vi "RRTPlan.vi"(4 "AttackerAvoidArea":bool=TRUE, 5 "Parameters.lvclass":refnum<class "Parameters.lvclass">, 6 "Line?":bool, 7 "Volta ao redor\nda área?":bool, 8 "Initial Pos x,y":dbl[](array[numeric]), 9 "Dest x,y":dbl[](array[numeric]), 10 "IA State":T1={"our_robots"=[], "enemy_robots"=[], "balls"=[], "geometry"={"line_width"=0, "field_length"=0, "field_width"=0, "boundary_width"=0, "referee_width"=0, "goal_width"=0, "goal_depth"=0, "goal_wall_width"=0, "center_circle_radius"=0, "defense_radius"=0, "defense_stretch"=0, "free_kick_from_defense_dist"=0, "penalty_spot_from_field_line_dist"=0, "penalty_line_from_spot_dist"=0}, "IA Judge"={"stage"="", "command"="", "our_goalie_id"=0.0, "enemy_goalie_id"=0.0, "command enum"=enum."Halt", "Time"=enum."Azul", "Point"={"x"=0.0, "y"=0.0}}, "Received Timestamp"=timestamp(0 s since 1904-01-01), "Events"={"Touch"=FALSE, "Ball out"=FALSE, "id touch"=0.0, "Ball out of \nVision"=FALSE, "Ball inside \nGoalie area"=FALSE, "Robot not responding"=FALSE, "Robots responding status"=[1.0, 1.0, 1.0, 1.0, 1.0, 1.0], "Enemy Ball \nPossession"=FALSE, "Pass State"=FALSE, "id end of pass"=0.0, "Kick"=FALSE, "Id ini Possession"=0.0, "Ball Possesion"=FALSE, "Id Possesion"=0.0, "Direct Kick"=FALSE, "2nd Strk Ativo"=FALSE}}, 11 "Robot":T2={"id"=0, "function"=enum."Attacker", "x"=0.0, "y"=0.0, "orientation"=0.0, "v_tangent"=0.0, "v_normal"=0.0, "v_ang"=0.0, "kick_x"=0.0, "kick_z"=0.0, "dribble"=FALSE, "Timestamp"=timestamp(0 s since 1904-01-01), "estimatives"={"est_v_tangent"=0.0, "est_v_normal"=0.0, "est_vx"=0.0, "est_vy"=0.0, "Pos Robot Est"=[], "est_v_ang"=0.0}, "dest_x_kick"=0.0, "dest_y_kick"=0.0, "Gap Coord"=[], "States"=enum."GoToTangent", "Path "=[], "Path  Smooth"=[], "Dest"=[], "vx_desired"=0.0, "vy_desired"=0.0, "slowBehavior"=FALSE, "VSSStates"=enum."Pass", "robotKickState"=enum."none", "role"=enum."DefenderArea"}) -> (0 "Path":dbl[][](array[numeric]), 1 "Smooth Path":dbl[][](array[numeric]))   [LabVIEW 2020]
uses:
  Vision_class/Old vision/Controls/AI Robot.ctl
  Vision_class/Old vision/Controls/Functions Enum.ctl
  Controls/estimatives.ctl
  Vision_class/Old vision/Controls/AttackerStates.ctl
  Vision_class/Old vision/Controls/PathDests.ctl
  Vision_class/Old vision/Controls/PathDest.ctl
  Navigation/VSSNavigation/VSSAttackerStates.ctl
  Robot_class/robotKickToStates.ctl
  Robot_class/roles.ctl
  Vision_class/Old vision/SSL Detection Frame Simple Estimator Cameras VelCmd Folder/Core/AI Input.ctl
  Vision_class/Old vision/SSL Detection Frame Simple Estimator Cameras VelCmd Folder/Core/AI Ball.ctl
  Vision_class/Old vision/SSL Detection Frame Simple Estimator Cameras VelCmd Folder/Core/Field Size.ctl
  Vision_class/Old vision/SSL Detection Frame Simple Estimator Cameras VelCmd Folder/Core/AI Judge.ctl
  Communication_class/Paths/MessageAI_State Folder/Intel/Command Enum.ctl
  Vision_class/Old vision/SSL Detection Frame Simple Estimator Cameras VelCmd Folder/Util/Events/Events.ctl
  Parameters_class/Parameters.lvclass
  Utilities_class/Utilities.lvclass
  Parameters_class/Parameters.lvclass/Parameters.ctl
  <vilib>/Analysis/_algsub.llb/Real Vector Norm.vi
  Parameters_class/Read Project.vi
  <vilib>/Analysis/NI_AALPro.lvlib
panel:
  in  "Path out":dbl[][](array[numeric])
  out "Path out 2":dbl[][](array[numeric])
  in  "WayPointProb":dbl=0.6 format="%#_13g"
  in  "GoalProb":dbl=0.1 format="%#_13g"
  in  "Step":dbl=80.0
  out "Goal":dbl[](array[numeric])
  out "Initial State":dbl[](array[numeric])
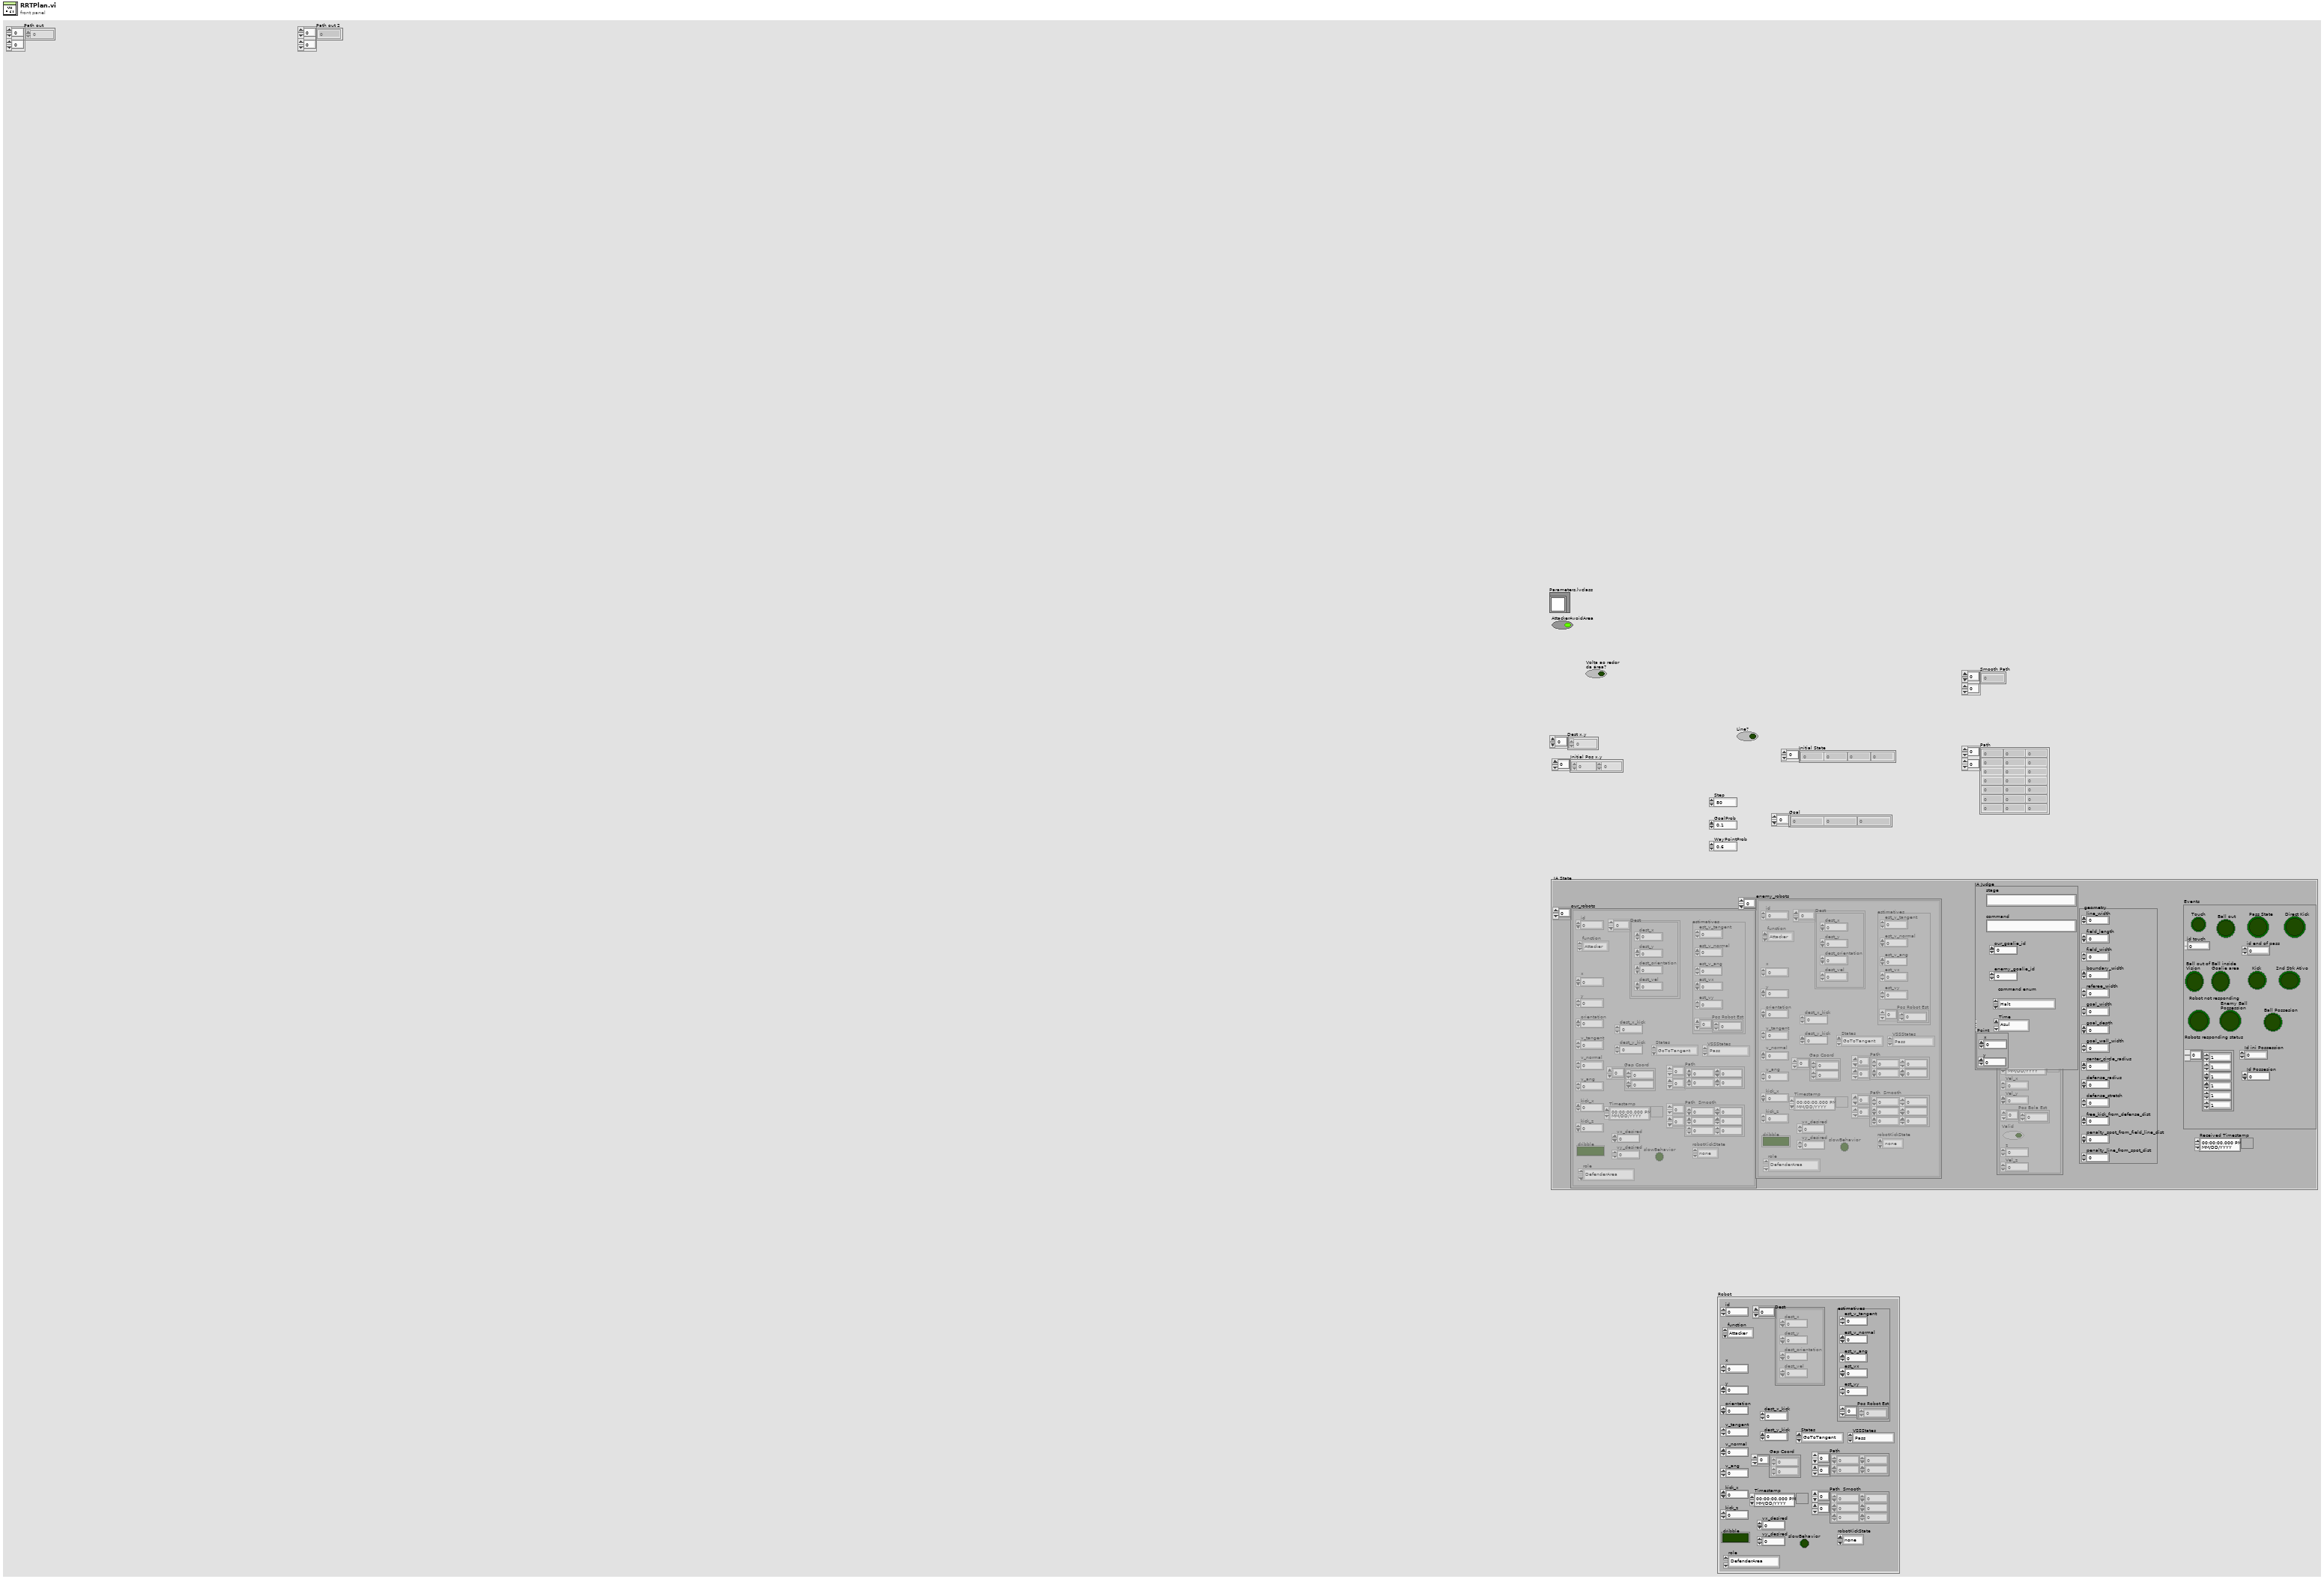
[diagram p1: front panel]
types:
  T1 = typedef "AI Input.ctl" = cluster{"our_robots":T2[], "enemy_robots":T2[], "balls":T11[], "geometry":T12, "IA Judge":T13, "Received Timestamp":timestamp, "Events":T15}
  T2 = typedef "AI Robot.ctl" = cluster{"id":u32, "function":T3, "x":dbl, "y":dbl, "orientation":dbl, "v_tangent":dbl, "v_normal":dbl, "v_ang":dbl, "kick_x":dbl, "kick_z":dbl, "dribble":bool, "Timestamp":timestamp, "estimatives":T4, "dest_x_kick":dbl, "dest_y_kick":dbl, "Gap Coord":dbl[], "States":T5, "Path ":dbl[][], "Path  Smooth":dbl[][], "Dest":T6, "vx_desired":dbl, "vy_desired":dbl, "slowBehavior":bool, "VSSStates":T8, "robotKickState":T9, "role":T10}
  T3 = typedef "Functions Enum.ctl" = enum16{"2nd Striker", "Attacker", "Goalie", "Defender", "Striker", "Goto 0", "Dummy", "Kicker", "ZigZag 0", "ZigZag 1", "ZigZag 2", "ZigZag 3", "ZigZag 4", "ZigZag 5", "ZigZag 6", "ZigZag 7", "ZigZag 8", ""}
  T4 = typedef "estimatives.ctl" = cluster{"est_v_tangent":dbl, "est_v_normal":dbl, "est_vx":dbl, "est_vy":dbl, "Pos Robot Est":dbl[], "est_v_ang":dbl}
  T5 = typedef "AttackerStates.ctl" = enum16{"Pass", "GoToTangent", "BallGetting", "GoToKick", ""}
  T6 = typedef "PathDests.ctl" = T7[]
  T7 = typedef "PathDest.ctl" = cluster{"dest_x":dbl, "dest_y":dbl, "dest_orientation":dbl, "dest_vel":dbl}
  T8 = typedef "VSSAttackerStates.ctl" = enum16{"Pass", "GoToTangent", "BallGetting", "GoToKick", "Rotate anti-clockwise", "Rotate Clockwise", ""}
  T9 = typedef "robotKickToStates.ctl" = enum16{"oldKickTo", "shootFromDirect", "avoidCollideBall", "goToBackBall", "none", "andar", "girar", "chutar"}
  T10 = typedef "roles.ctl" = enum16{"SecondMarker", "5Robots5th", "PassBestReceiver", "5Robots4th", "5Robots3rd", "5Robots2nd", "5Robots1st", "PassBestRobot", "WaitPass", "ABCThirdKicker", "ABCFirstKicker", "ABCSecondKicker", "Tabler", "TableFinalizer", "PrepareRollToPassRoller", "PrepareRollToPassReceiver", "SimplePassRoll", "SimplePassRollReceiver", "PenaltyDefense", "PreparePassReceiver 2", "PreparePassReceiver 1", "PassObserver", "Timeout", "Goto", "ZigZag", "None", "BallOutOfField", "DefenderArea", "Duelist", "AttackerStop", "FollowAttacker", "KeeperRole", "KickPenalty", "AttackerAimGoal", "AttackerBlock", "Marker", "Halt", "Shoot", "PassKicker", "PassReceiver", "TestRole", "PenaltyAttacker"}
  T11 = typedef "AI Ball.ctl" = cluster{"x":dbl, "y":dbl, "timestamp":timestamp, "Vel_x":dbl, "Vel_y":dbl, "Pos Bola Est":dbl[], "Valid":bool, "z":dbl, "Vel_z":dbl}
  T12 = typedef "Field Size.ctl" = cluster{"line_width":u32, "field_length":u32, "field_width":u32, "boundary_width":u32, "referee_width":u32, "goal_width":u32, "goal_depth":u32, "goal_wall_width":u32, "center_circle_radius":u32, "defense_radius":u32, "defense_stretch":u32, "free_kick_from_defense_dist":u32, "penalty_spot_from_field_line_dist":u32, "penalty_line_from_spot_dist":u32}
  T13 = typedef "AI Judge.ctl" = cluster{"stage":string, "command":string, "our_goalie_id":dbl, "enemy_goalie_id":dbl, "command enum":T14, "Time":enum16{"Azul", "Amarelo"}, "Point":cluster{"x":sgl, "y":sgl}}
  T14 = typedef "Command Enum.ctl" = enum16{"Halt", "Stop", "Force Start", "PKA Normal Start", "Prepare Kickoff Ally", "PKE Normal Start", "Prepare Kickoff Enemy", "Prepare Penalty Ally", "PPA Normal Start", "Prepare Penalty Enemy", "PPE Normal Start", "Direct Free Enemy", "Direct Free Ally", "Indirect Free Enemy", "Indirect Free Ally", "Timeout Enemy", "Timeout Ally", "Goal Enemy", "Goal Ally", "Ball Placement Enemy", "Ball Placement Ally", "Normal Half Time", "Extra Time Break", "Extra Half Time", "None", "Post Game"}
  T15 = typedef "Events.ctl" = cluster{"Touch":bool, "Ball out":bool, "id touch":dbl, "Ball out of \nVision":bool, "Ball inside \nGoalie area":bool, "Robot not responding":bool, "Robots responding status":dbl[], "Enemy Ball \nPossession":bool, "Pass State":bool, "id end of pass":dbl, "Kick":bool, "Id ini Possession":dbl, "Ball Possesion":bool, "Id Possesion":dbl, "Direct Kick":bool, "2nd Strk Ativo":bool}
  T16 = typedef "Project.ctl" = enum16{"SSL", "VSS"}
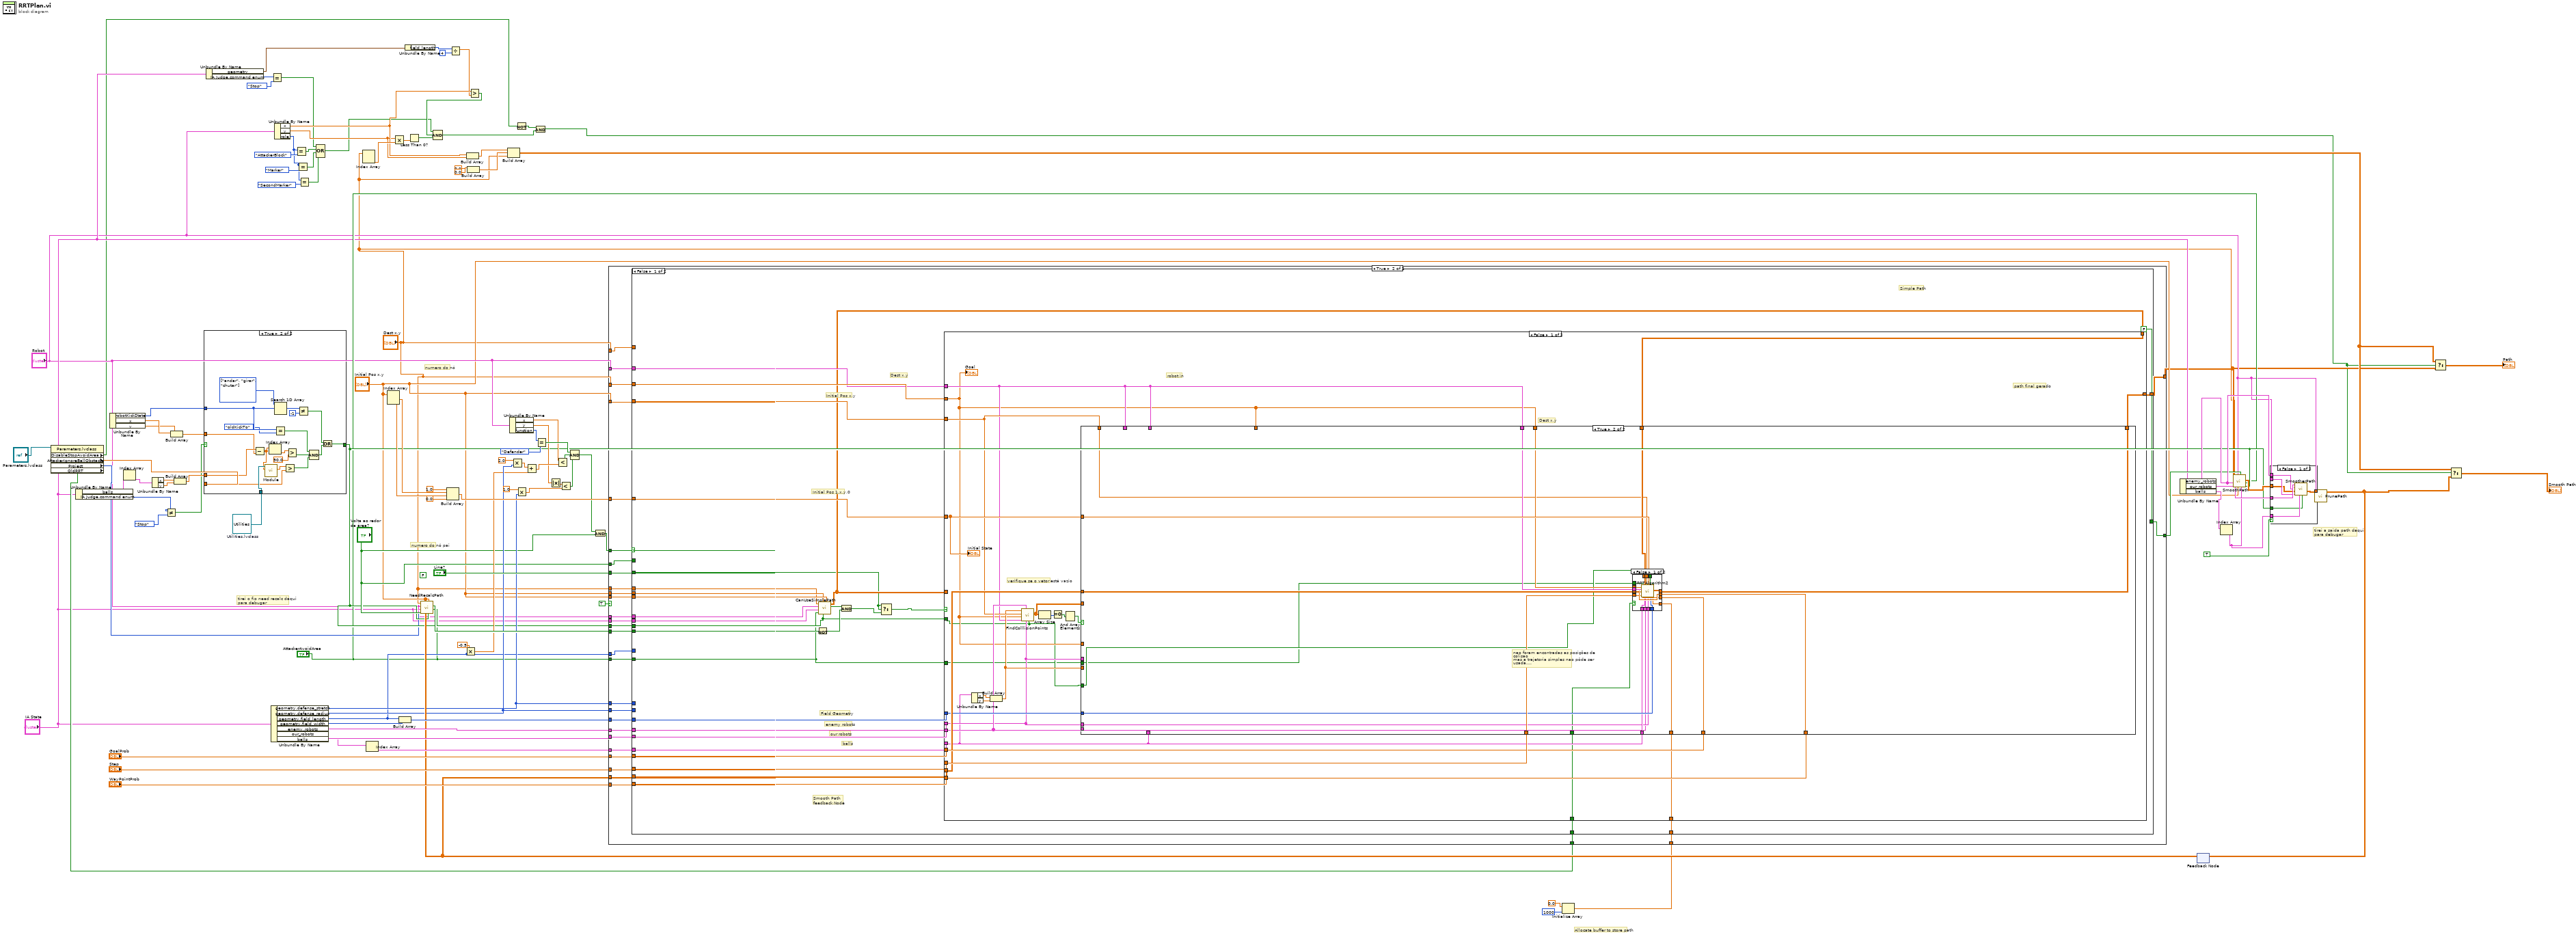
[diagram p0: block diagram]
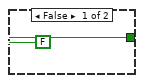
[diagram p2: hidden frame]
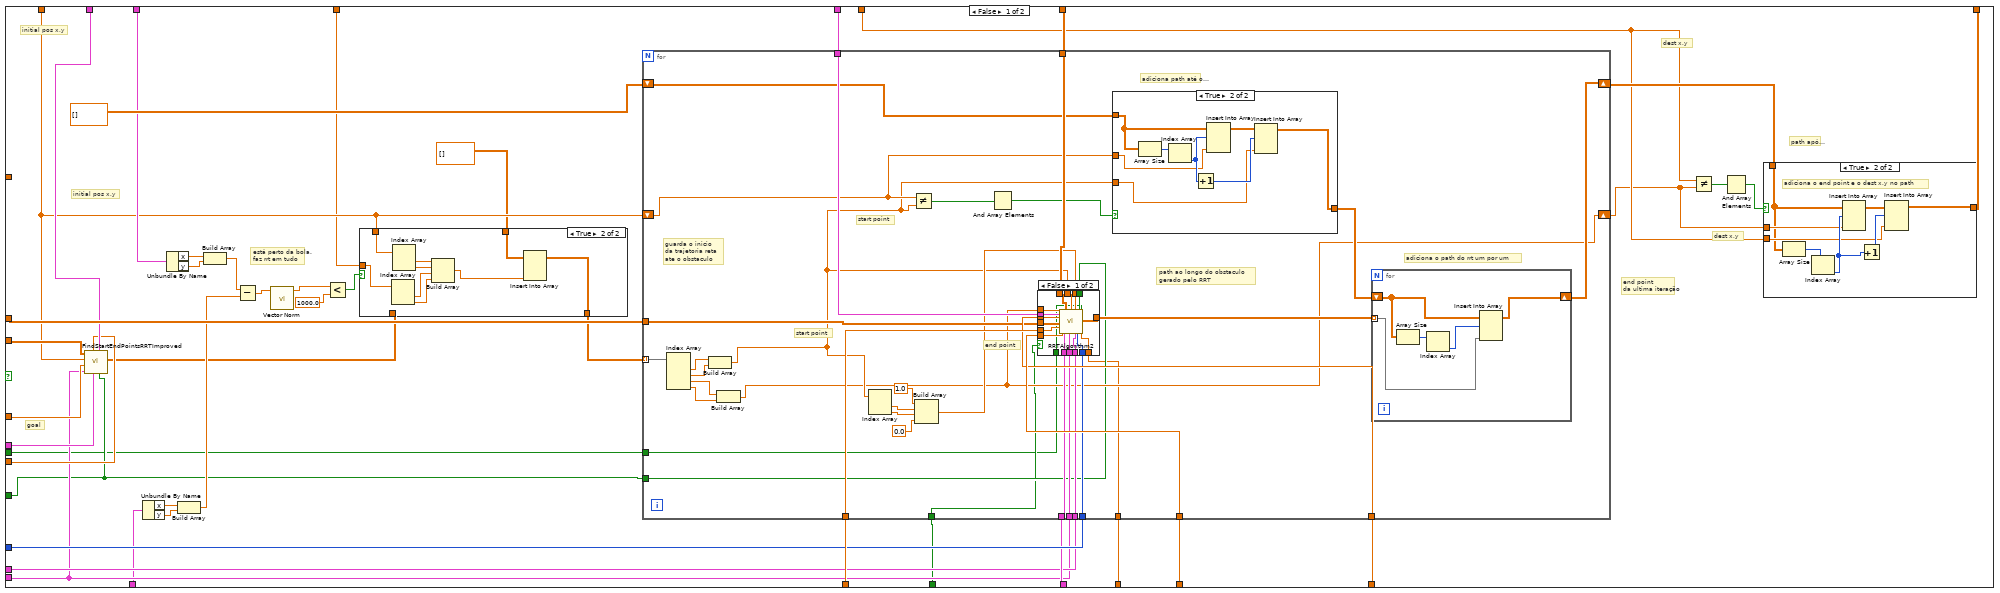
[diagram p4: hidden frame]
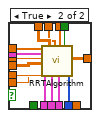
[diagram p7: hidden frame]
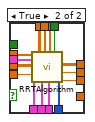
[diagram p9: hidden frame]
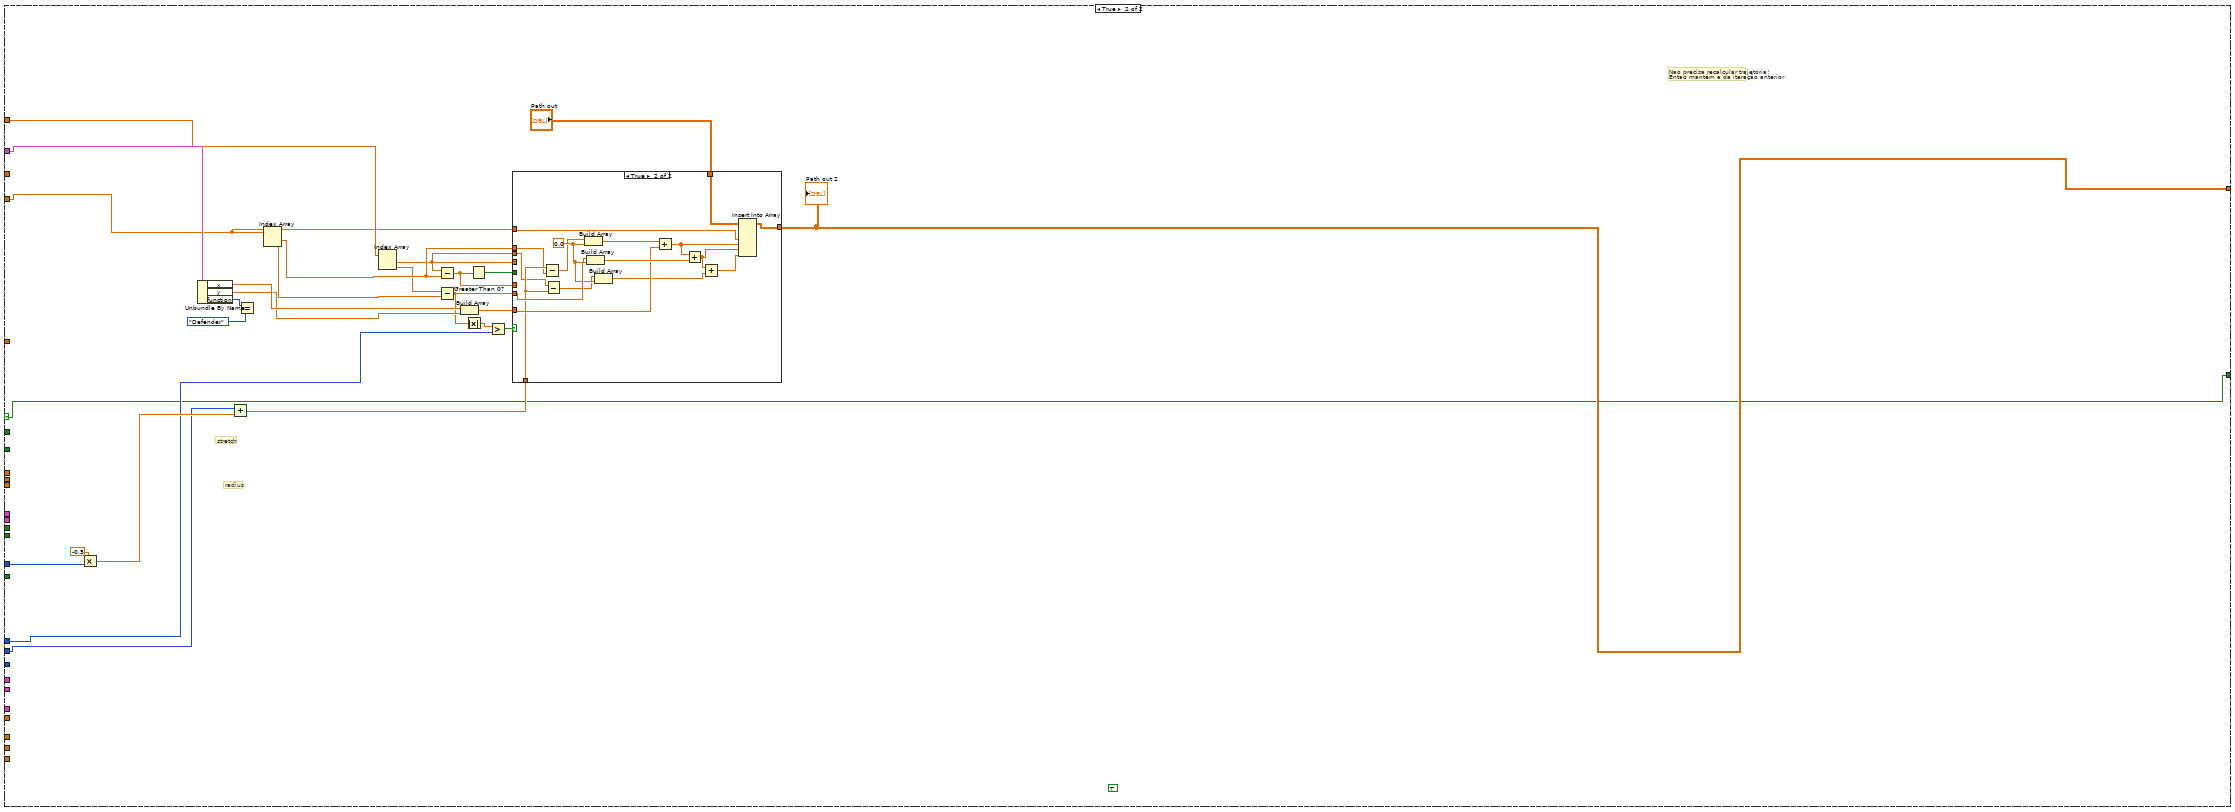
[diagram p11: hidden frame]
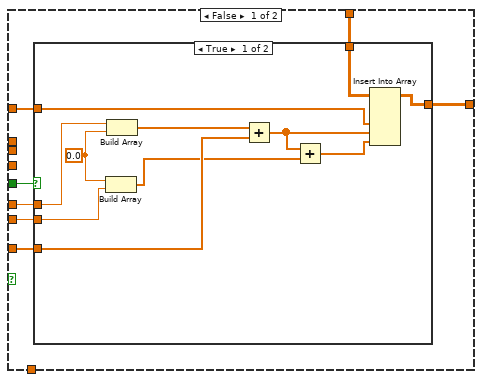
[diagram p12: hidden frame]
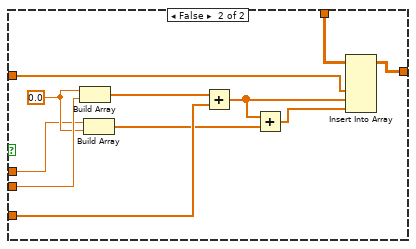
[diagram p13: hidden frame]
diagram:
  w51 = refnum<class "Utilities.lvclass"> refnum  # Utilities.lvclass
  (unwired) FALSE
  # "Allocate buffer to store path"
  # "tirei a saida path daqui\npara debugar"
  # "tirei o fio need recalc daqui\npara debugar"
  # "numero do nó pai"
  # "numero do nó"
  n1 = property class="Parameters.lvclass"(reference="Parameters.lvclass") -> ("DisableStopAvoidArea"=w3:bool, "AttackerIgnoreBallObstacle"=w49:dbl, "Project"=w47:T16, "OldRRT"=w46:bool)  [unwired: 1 in, 2 out]
  n2 = Unbundle By Name("IA State") -> ("balls"=w59:T11[], "IA Judge.command enum"=w55:T14)
  n3 = Unbundle By Name("Robot") -> ("robotKickState"=w42:T9, "x"=w61:dbl, "y"=w60:dbl)
  n4 = Index Array(array=w59) -> (element=w58:T11)  [unwired: 1 in]
  n5 = Unbundle By Name(w58) -> ("x"=w57:dbl, "y"=w56:dbl)
  n6 = Not Equal?(x=w55, y=Command_Enum."Stop" ("IA Judge.command enum")) -> (x != y?=w41:bool)
  n7 = Build Array(w61, w60) -> (w53:dbl[])
  n8 = Build Array(w57, w56) -> (w52:dbl[])
  n9 = case shown="True" w41 {
    tunnel: w53 -> [_ w126]
    tunnel: w52 -> [_ w127]
    tunnel: [FALSE w117] -> w48
    tunnel: w51 -> [_ w125]
    tunnel: w49 -> [_ w121]
    tunnel: w42 -> [_ w111]
    frame False {
    }
    frame True {
      w115 = T9[] [enum."andar", enum."girar", enum."chutar"] items=["oldKickTo", "shootFromDirect", "avoidCollideBall", "goToBackBall", "none", "andar", "girar", "chutar"] ("1D array")
      n10 = Subtract(x=w127, y=w126) -> (x-y=w124:dbl[])
      n11 = call "Module.vi"("2D vector"=w124, "Utilities in"=w125) -> ("Modulo"=w123:dbl)  [unwired: 7 in, 2 out]
      n12 = Index Array(array=w124) -> (element=w120:dbl)  [unwired: 1 in]
      n13 = Equal?(x=w111, y=robotKickToStates."oldKickTo") -> (x = y?=w109:bool)
      n14 = Search 1D Array(1D array=w115, element=w111) -> (index of element=w114:i32)  [unwired: 1 in]
      n15 = Greater?(x=w123, y=w121) -> (0:w122:bool)
      n16 = Greater?(x=w120, y=90.0) -> (0:w118:bool)
      n17 = Not Equal?(x=w114, y=-1) -> (x != y?=w112:bool)
      n18 = Compound Arithmetic op=AND(w109, w118, w122) -> (w116:bool)
      n19 = Or(x=w112, y=w116) -> (x .or. y?=w117:bool)
    }
  }
  n20 = Unbundle By Name("IA State") -> ("geometry"=w23:T12, "IA Judge.command enum"=w37:T14)
  n21 = Unbundle By Name("IA State") -> ("geometry.defense_stretch"=w69:u32, "geometry.defense_radius"=w68:u32, "geometry.field_length"=w66:u32, "geometry.field_width"=w84:u32, "enemy_robots"=w103:T2[], "our_robots"=w100:T2[], "balls"=w96:T11[])
  n22 = Equal?(x=w37, y=Command_Enum."Stop") -> (x = y?=w6:bool)
  n23 = Unbundle By Name("Robot") -> ("x"=w20:dbl, "y"=w15:dbl, "role"=w11:T10)
  n24 = Equal?(x=w11, y=roles."AttackerBlock" ("role")) -> (x = y?=w10:bool)
  n25 = Equal?(x=w11, y=roles."Marker" ("role")) -> (x = y?=w9:bool)
  n26 = Equal?(x=w11, y=roles."SecondMarker" ("role")) -> (x = y?=w8:bool)
  n27 = Compound Arithmetic op=OR(w6, w10, w9, w8) -> (w5:bool)
  n28 = Index Array(array="Dest x,y") -> (element #2=w31:dbl)  [unwired: 2 in, 1 out]
  n29 = Index Array(array=w96) -> (element=w95:T11)  [unwired: 1 in]
  n30 = Index Array(array="Initial Pos x,y") -> (element #1=w99:dbl, element #2=w98:dbl)  [unwired: 2 in]
  n31 = Multiply(x=w15, y=w31) -> (x*y=w33:dbl)
  n32 = Build Array(w66, w84) -> (w107:u32[])
  n33 = Unbundle By Name(w23) -> ("field_length"=w22:u32)
  n34 = Less Than 0?(x=w33) -> (x < 0?=w32:bool)
  n35 = Build Array(1.0 ("element"), w99, w98, 0.0 ("element")) -> (w93:dbl[])
  n36 = Divide(x=w22, y=u32 4) -> (x/y=w19:dbl)
  n37 = Multiply(x=-0.5, y=w66) -> (x*y=w65:dbl)
  n38 = Build Array(w20, w15) -> (w16:dbl[])
  n39 = Build Array(0.0 ("element"), 0.0 ("element")) -> (w18:dbl[])
  n40 = Greater?(x=w20, y=w19) -> (0:w7:bool)
  n41 = Compound Arithmetic op=AND(w5, w7, w32) -> (w2:bool)
  n42 = Build Array(w16, w18, "Dest x,y") -> (w26:dbl[][])
  n43 = Unbundle By Name("Robot") -> ("x"=w71:dbl, "y"=w70:dbl, "function"=w82:T3)
  n44 = Multiply(x=2.0, y=w68) -> (x*y=w79:dbl)
  n45 = Not(x=w3) -> (.not. x?=w4:bool)
  n46 = Multiply(x=1.0, y=w69) -> (x*y=w73:dbl)
  n47 = Add(x=w79, y=w65) -> (x+y=w78:dbl)
  n48 = And(x=w4, y=w2) -> (x .and. y?=w1:bool)
  n49 = Equal?(x=w82, y=Functions_Enum."Defender") -> (x = y?=w76:bool)
  n50 = Absolute Value(x=w70) -> (abs(x)=w75:dbl)
  n51 = Less?(x=w71, y=w78) -> (x < y?=w77:bool)
  n52 = Less?(x=w75, y=w73) -> (x < y?=w72:bool)
  n53 = Compound Arithmetic op=AND(w76, w77, w72) -> (w64:bool)
  n54 = And(x=w64, y="Volta ao redor\nda área?") -> (x .and. y?=w62:bool)
  n55 = Initialize Array(0.0, 1000) -> (w43:dbl[])
  n56 = Unbundle By Name("IA State") -> ("enemy_robots"=w89:T2[], "our_robots"=w90:T2[], "balls"=w97:T11[])
  n57 = feedback #1() -> (w94:dbl[][])  [unwired: 1 in]
  n58 = call "NeedRecalcPath.vi"("Project"=w47, "AttackerAvoidArea"="AttackerAvoidArea", "ignoreBall?"=w48, "Initial State"="Initial Pos x,y", "SmoothPath"=w94, "Pos x,y"="Initial Pos x,y", "Volta ao redor\nda área?"="Volta ao redor\nda área?", "IA State"="IA State", "Robot"="Robot", "Dest x,y"="Dest x,y") -> ("result"=w92:bool)  [unwired: 1 out]
  n59 = case shown="True" TRUE {
    tunnel: w107 -> [_ w160]
    tunnel: "Step" -> [_ w159]
    tunnel: "GoalProb" -> [_ w158]
    tunnel: "WayPointProb" -> [_ w157]
    tunnel: w103 -> [_ w156]
    tunnel: w93 -> [_ w155]
    tunnel: w94 -> [w129 w154]
    tunnel: w100 -> [_ w153]
    tunnel: [w129 w152] -> w25
    tunnel: "Dest x,y" -> [_ w151]
    tunnel: "Initial Pos x,y" -> [_ w150]
    tunnel: "Robot" -> [_ w149]
    tunnel: w95 -> [_ w148]
    tunnel: "Initial Pos x,y" -> [_ w147]
    tunnel: "Initial Pos x,y" -> [_ w146]
    tunnel: "Dest x,y" -> [_ w145]
    tunnel: "Robot" -> [_ w144]
    tunnel: "IA State" -> [_ w143]
    tunnel: w92 -> [_ w142]
    tunnel: w69 -> [_ w138]
    tunnel: w68 -> [_ w137]
    tunnel: "Dest x,y" -> [_ w134]
    tunnel: w66 -> [_ w136]
    tunnel: [w128 w141] -> w85
    tunnel: "Line?" -> [_ w140]
    tunnel: "Volta ao redor\nda área?" -> [_ w135]
    tunnel: w62 -> [w128 w139]
    tunnel: w48 -> [_ w133]
    tunnel: w46 -> [_ w132]
    tunnel: w43 -> [_ w131]
    tunnel: "AttackerAvoidArea" -> [_ w130]
    frame False {
    }
    frame True {
      n60 = case shown="False" w139 {
        selector: w139 -> [_ w408]
        tunnel: w160 -> [w190 _]
        tunnel: w159 -> [w189 _]
        tunnel: w158 -> [w188 _]
        tunnel: w157 -> [w187 _]
        tunnel: w156 -> [w186 _]
        tunnel: w155 -> [w185 _]
        tunnel: w154 -> [w184 _]
        tunnel: w153 -> [w183 _]
        tunnel: [w182 w418] -> w152
        tunnel: w151 -> [w181 _]
        tunnel: w150 -> [w180 w419]
        tunnel: w149 -> [w179 w421]
        tunnel: w148 -> [w178 _]
        tunnel: w147 -> [w177 _]
        tunnel: w146 -> [w176 _]
        tunnel: w145 -> [w175 _]
        tunnel: w144 -> [w174 _]
        tunnel: w143 -> [w173 _]
        tunnel: w142 -> [w171 _]
        tunnel: [FALSE w408] -> w141
        tunnel: w140 -> [w166 _]
        tunnel: w138 -> [_ w424]
        tunnel: w137 -> [_ w423]
        tunnel: w136 -> [_ w422]
        tunnel: w135 -> [_ _]
        tunnel: w134 -> [_ w420]
        tunnel: w133 -> [w164 _]
        tunnel: w132 -> [w163 _]
        tunnel: w131 -> [w162 _]
        tunnel: w130 -> [w161 _]
        frame False {
          # "Initial Pos 1,x,y,0"
          # "Initial Pos x,y"
          # "Dest x,y"
          # "Simple Path"
          # "balls"
          # "our robots"
          # "enemy robots"
          # "Field Geometry"
          # "Smooth Path \nfeedback Node"
          n61 = Not(x=w171) -> (.not. x?=w170:bool)
          n62 = call "CanUseSimplePath.vi"("Initial State"=w177, "ignoreBall?"=w164, "Pos x,y"=w176, "AttackerAvoidArea"=w161, "IA State"=w173, "Robot"=w174, "Dest x,y"=w175) -> (2:"Simple Path"=w172:bool, 3:"Simple Path"=w169:dbl[][])  [unwired: 3 in]
          n63 = And(x=w172, y=w170) -> (x .and. y?=w167:bool)
          n64 = Select(t=w166, s=w166, f=w167) -> (s? t:f=w168:bool)
          n65 = case shown="False" w168 {
            tunnel: w190 -> [w211 _]
            tunnel: w189 -> [w215 _]
            tunnel: w179 -> [w197 _]
            tunnel: w188 -> [w214 _]
            tunnel: w187 -> [w213 _]
            tunnel: w186 -> [w198 _]
            tunnel: w184 -> [w212 _]
            tunnel: [w208 w407] -> w182
            tunnel: w181 -> [w195 _]
            tunnel: w180 -> [w200 _]
            tunnel: w185 -> [w210 _]
            tunnel: w183 -> [w205 _]
            tunnel: w178 -> [w196 _]
            tunnel: w169 -> [_ w407]
            tunnel: w169 -> [w209 _]
            tunnel: w164 -> [w194 _]
            tunnel: w163 -> [w193 _]
            tunnel: w162 -> [w192 _]
            tunnel: w161 -> [w191 _]
            frame False {
              # "robot in"
              # "path final gerado"
              # "Dest x,y"
              # "verifique se o vetor está vazio"
              n66 = Unbundle By Name(w196) -> ("x"=w207:dbl, "y"=w206:dbl)
              n67 = Build Array(w207, w206) -> (w199:dbl[])
              n68 = call "FindColllisionPoints.vi"("ignoreBall?"=w194, "enemy_robots"=w198, "our_robots"=w205, "Robot in"=w197, "Goal"=w195, "Initial State"=w200, "ball"=w199) -> ("Collision Points"=w201:dbl[][])  [unwired: 4 in]
              n69 = Array Size(array=w201) -> (size(s)=w204:i32[])
              n70 = Equal To 0?(x=w204) -> (x = 0?=w202:bool[])
              n71 = And Array Elements(Boolean array=w202) -> (logical AND=w203:bool)
              n72 = case shown="True" w203 {
                tunnel: w215 -> [w258 w374]
                tunnel: w214 -> [w257 w373]
                tunnel: w213 -> [w256 w372]
                tunnel: w212 -> [w255 w371]
                tunnel: w211 -> [w254 w370]
                tunnel: w210 -> [_ w369]
                tunnel: w209 -> [w253 w368]
                tunnel: [w243 w367] -> w208
                tunnel: w196 -> [w252 w366]
                tunnel: w195 -> [w242 w365]
                tunnel: w197 -> [w251 w364]
                tunnel: w198 -> [w250 w363]
                tunnel: w205 -> [w237 w362]
                tunnel: w201 -> [w249 _]
                tunnel: w200 -> [w222 w361]
                tunnel: w195 -> [w248 _]
                tunnel: w197 -> [w240 _]
                tunnel: w199 -> [w239 _]
                tunnel: w198 -> [w238 _]
                tunnel: w197 -> [w236 _]
                tunnel: w196 -> [w235 _]
                tunnel: w195 -> [w221 _]
                tunnel: w194 -> [w219 w360]
                tunnel: w193 -> [w218 w359]
                tunnel: w192 -> [w217 w358]
                tunnel: w191 -> [w216 w357]
                frame False {
                  # "está perto da bola.\nfaz rrt em tudo"
                  # "dest x,y"
                  # "end point \nda ultima iteração"
                  # "dest x,y"
                  # "path após RRT até o destino final"
                  # "initial pos x,y"
                  # "initial pos x,y"
                  # "goal"
                  n73 = call "FindStartEndPointsRRTImproved.vi"("ignoreBall?"=w219, "Robot in"=w240, "enemy_robots"=w238, "ball"=w239, "our_robots"=w237, "Goal"=w248, "Initial State"=w222, "Collision Points"=w249) -> ("Start End Points RRT"=w224:dbl[][])  [unwired: 3 in]
                  n74 = Unbundle By Name(w235) -> ("x"=w232:dbl, "y"=w231:dbl)
                  n75 = Unbundle By Name(w236) -> ("x"=w234:dbl, "y"=w233:dbl)
                  n76 = Build Array(w232, w231) -> (w229:dbl[])
                  n77 = Build Array(w234, w233) -> (w230:dbl[])
                  n78 = Subtract(x=w230, y=w229) -> (x-y=w228:dbl[])
                  n79 = call-poly <vilib>:"Vector Norm.vi"("Input Vector"=w228) -> ("norm"=w227:dbl)  [unwired: 9 in, 1 out]
                  n80 = Less?(x=w227, y=1000.0) -> (x < y?=w225:bool)
                  n81 = case shown="True" w225 {
                    tunnel: [w259 w260] -> w223
                    tunnel: w224 -> [w259 _]
                    tunnel: w222 -> [_ w268]
                    tunnel: w221 -> [_ w265]
                    tunnel: dbl[][] [] -> [_ w262]
                    frame False {
                    }
                    frame True {
                      n82 = Index Array(array=w265) -> (element #1=w264:dbl, element #2=w263:dbl)  [unwired: 2 in]
                      n83 = Index Array(array=w268) -> (element #1=w267:dbl, element #2=w266:dbl)  [unwired: 2 in]
                      n84 = Build Array(w267, w266, w264, w263) -> (w261:dbl[])
                      n85 = Insert Into Array(array=w262, new element=w261) -> (w260:dbl[][])  [unwired: 2 in]
                    }
                  }
                  n86 = for {
                    tunnel: w258 -> [w310]
                    tunnel: w257 -> [w309]
                    tunnel: w256 -> [w308]
                    tunnel: w255 -> [w307]
                    tunnel: w254 -> [w306]
                    tunnel: w253 -> [w305]
                    tunnel: w252 -> [w304]
                    tunnel: w251 -> [w303]
                    tunnel: w250 -> [w302]
                    tunnel: w237 -> [w301]
                    tunnel: w223 -> [w291] mode=indexing
                    shift-right: [w282] -> w241
                    shift-left: w222 -> [w285]
                    shift-right: [w283] -> w244
                    shift-left: dbl[][] [] -> [w286]
                    tunnel: w219 -> [w281]
                    tunnel: w218 -> [w280]
                    tunnel: w217 -> [w279]
                    tunnel: w216 -> [w278]
                    # "adiciona o path do rrt um por um"
                    # "start point"
                    # "guarda o inicio\nda trajetoria reta\nate o obstaculo"
                    # "end point"
                    # "start point"
                    # "path ao longo do obstaculo\ngerado pelo RRT"
                    # "adiciona path até o obstaculo"
                    n87 = Index Array(array=w291) -> (element #1=w290:dbl, element #2=w289:dbl, element #3=w288:dbl, element #4=w287:dbl)  [unwired: 4 in]
                    n88 = Build Array(w290, w289) -> (w284:dbl[])
                    n89 = Build Array(w288, w287) -> (w282:dbl[])
                    n90 = Index Array(array=w284) -> (element #1=w298:dbl, element #2=w297:dbl)  [unwired: 2 in]
                    n91 = Not Equal?(x=w285, y=w284) -> (x != y?=w294:bool[])
                    n92 = Build Array(1.0 ("element"), w298, w297, 0.0 ("element")) -> (w296:dbl[])
                    n93 = And Array Elements(Boolean array=w294) -> (logical AND=w293:bool)
                    n94 = case shown="False" w280 {
                      tunnel: w310 -> [w317 w342]
                      tunnel: w309 -> [w318 w341]
                      tunnel: w308 -> [w315 w340]
                      tunnel: w307 -> [w316 w339]
                      tunnel: w306 -> [w322 w338]
                      tunnel: w305 -> [w323 w337]
                      tunnel: w304 -> [w319 w336]
                      tunnel: w303 -> [w314 w335]
                      tunnel: w302 -> [w321 w334]
                      tunnel: w301 -> [w320 w333]
                      tunnel: w296 -> [w325 w332]
                      tunnel: [w327 w331] -> w295
                      tunnel: w284 -> [w324 w330]
                      tunnel: w282 -> [w313 w329]
                      tunnel: w281 -> [w326 w328]
                      tunnel: w279 -> [w312 _]
                      tunnel: w278 -> [w311 _]
                      frame False {
                        n95 = call "RRTAlgorithm2.vi"("Dest x,y"=w313, "Robot"=w314, "WayPointProb"=w315, "Path in \n(Smooth do Feedback Node)"=w316, "Step"=w317, "GoalProb"=w318, "Simple Path"=w323, "Ball"=w319, "Initial Pos x,y"=w324, "our_robots"=w320, "Initial Pos 1,x,y,0"=w325, "enemy_robots"=w321, "ignoreBall?"=w326, "Field Geomtery"=w322, "AttackerAvoidArea"=w311, "buffer"=w312) -> ("Path"=w327:dbl[][])  [unwired: 3 in]
                      }
                      frame True {
                        n96 = call "RRTAlgorithm.vi"("Dest x,y"=w329, "Robot"=w335, "WayPointProb"=w340, "Path in \n(Smooth do Feedback Node)"=w339, "Step"=w342, "GoalProb"=w341, "Simple Path"=w337, "Ball"=w336, "Initial Pos x,y"=w330, "our_robots"=w333, "Initial Pos 1,x,y,0"=w332, "enemy_robots"=w334, "ignoreBall?"=w328, "Field Geomtery"=w338) -> ("Path"=w331:dbl[][])  [unwired: 5 in]
                      }
                    }
                    n97 = case shown="True" w293 {
                      tunnel: [w343 w348] -> w292
                      tunnel: w286 -> [w343 w350]
                      tunnel: w285 -> [_ w345]
                      tunnel: w284 -> [_ w344]
                      frame False {
                      }
                      frame True {
                        n98 = Array Size(array=w350) -> (size(s)=w351:i32[])
                        n99 = Index Array(array=w351) -> (element=w347:i32)  [unwired: 1 in]
                        n100 = Increment(x=w347) -> (x+1=w346:i32)
                        n101 = Insert Into Array(array=w350, index (row)=w347, new element=w345) -> (w349:dbl[][])  [unwired: 1 in]
                        n102 = Insert Into Array(array=w349, index (row)=w346, new element=w344) -> (w348:dbl[][])  [unwired: 1 in]
                      }
                    }
                    n103 = for {
                      tunnel: w295 -> [w355] mode=indexing
                      shift-right: [w354] -> w283
                      shift-left: w292 -> [w356]
                      n104 = Array Size(array=w356) -> (size(s)=w353:i32[])
                      n105 = Index Array(array=w353) -> (element=w352:i32)  [unwired: 1 in]
                      n106 = Insert Into Array(array=w356, index (row)=w352, new element=w355) -> (w354:dbl[][])  [unwired: 1 in]
                    }
                  }
                  n107 = Not Equal?(x=w242, y=w241) -> (x != y?=w246:bool[])
                  n108 = And Array Elements(Boolean array=w246) -> (logical AND=w245:bool)
                  n109 = case shown="True" w245 {
                    tunnel: [w269 w271] -> w243
                    tunnel: w242 -> [_ w273]
                    tunnel: w241 -> [_ w272]
                    tunnel: w244 -> [w269 w270]
                    frame False {
                    }
                    frame True {
                      # "adiciona o end point e o dest x,y no path"
                      n110 = Array Size(array=w270) -> (size(s)=w277:i32[])
                      n111 = Index Array(array=w277) -> (element=w275:i32)  [unwired: 1 in]
                      n112 = Insert Into Array(array=w270, index (row)=w275, new element=w272) -> (w276:dbl[][])  [unwired: 1 in]
                      n113 = Increment(x=w275) -> (x+1=w274:i32)
                      n114 = Insert Into Array(array=w276, index (row)=w274, new element=w273) -> (w271:dbl[][])  [unwired: 1 in]
                    }
                  }
                }
                frame True {
                  # "nao foram encontradas as posições de colisao\nmas a trajetoria simples nao pôde ser usada.\nIncoerência, a princípio nunca vai cair nesse caso.\nCaso aconteça, aplique o RRT sobre toda a extensão."
                  n115 = case shown="False" w359 {
                    tunnel: w374 -> [w385 w406]
                    tunnel: w373 -> [w386 w405]
                    tunnel: w372 -> [w388 w404]
                    tunnel: w371 -> [w387 w403]
                    tunnel: w370 -> [w384 w402]
                    tunnel: w369 -> [w379 w401]
                    tunnel: w368 -> [w377 w400]
                    tunnel: [w391 w399] -> w367
                    tunnel: w366 -> [w381 w398]
                    tunnel: w365 -> [w390 w397]
                    tunnel: w364 -> [w389 w396]
                    tunnel: w363 -> [w383 w395]
                    tunnel: w362 -> [w382 w394]
                    tunnel: w361 -> [w378 w393]
                    tunnel: w360 -> [w380 w392]
                    tunnel: w358 -> [w376 _]
                    tunnel: w357 -> [w375 _]
                    frame False {
                      n116 = call "RRTAlgorithm2.vi"("Dest x,y"=w390, "Robot"=w389, "WayPointProb"=w388, "Path in \n(Smooth do Feedback Node)"=w387, "Step"=w385, "GoalProb"=w386, "Simple Path"=w377, "Ball"=w381, "Initial Pos x,y"=w378, "our_robots"=w382, "Initial Pos 1,x,y,0"=w379, "enemy_robots"=w383, "ignoreBall?"=w380, "Field Geomtery"=w384, "AttackerAvoidArea"=w375, "buffer"=w376) -> ("Path"=w391:dbl[][])  [unwired: 3 in]
                    }
                    frame True {
                      n117 = call "RRTAlgorithm.vi"("Dest x,y"=w397, "Robot"=w396, "WayPointProb"=w404, "Path in \n(Smooth do Feedback Node)"=w403, "Step"=w406, "GoalProb"=w405, "Simple Path"=w400, "Ball"=w398, "Initial Pos x,y"=w393, "our_robots"=w394, "Initial Pos 1,x,y,0"=w401, "enemy_robots"=w395, "ignoreBall?"=w392, "Field Geomtery"=w402) -> ("Path"=w399:dbl[][])  [unwired: 5 in]
                    }
                  }
                }
              }
              "Initial State" <- w210
              "Goal" <- w195
            }
            frame True {
              # "Pode usar a trajetória simples (reta) entre o estado inicial e o destino.\nAlém disso, nao precisa recalcular a trajetória."
            }
          }
        }
        frame True {
          (unwired) TRUE
          # "radius"
          # "stretch"
          # "Nao precisa recalcular trajetória!\nEntao mantém a da iteração anterior"
          n118 = Multiply(x=-0.5, y=w422) -> (x*y=w426:dbl)
          n119 = Unbundle By Name(w421) -> ("x"=w431:dbl, "y"=w427:dbl, "function"=w433:T3)
          n120 = Add(x=w423, y=w426) -> (x+y=w425:dbl)
          n121 = Equal?(x=w433, y=Functions_Enum."Defender") -> ()  [unwired: 1 out]
          n122 = Index Array(array=w419) -> (element #1=w429:dbl, element #2=w428:dbl)  [unwired: 2 in]
          n123 = Index Array(array=w420) -> (element #1=w411:dbl, element #2=w417:dbl)  [unwired: 2 in]
          n124 = Subtract(x=w411, y=w429) -> (x-y=w415:dbl)
          n125 = Subtract(x=w417, y=w428) -> (x-y=w409:dbl)
          n126 = Build Array(w431, w427) -> (w413:dbl[])
          n127 = Absolute Value(x=w409) -> (abs(x)=w410:dbl)
          n128 = Greater Than 0?(x=w415) -> (x > 0?=w416:bool)
          n129 = Greater?(x=w410, y=w424) -> (0:w412:bool)
          n130 = case shown="True" w412 {
            tunnel: w416 -> [w440 _]
            tunnel: w415 -> [w439 _]
            tunnel: "Path out" -> [w438 w475]
            tunnel: [w437 w476] -> w418
            tunnel: w413 -> [w436 w473]
            tunnel: w419 -> [w435 w474]
            tunnel: w409 -> [w434 w469]
            tunnel: w425 -> [_ w466]
            tunnel: w411 -> [_ _]
            tunnel: w411 -> [_ w465]
            tunnel: w429 -> [_ w463]
            frame False {
              n131 = case shown="True" w440 {
                tunnel: w439 -> [w448 w459]
                tunnel: w434 -> [w450 w461]
                tunnel: w438 -> [w451 w462]
                tunnel: [w447 w458] -> w437
                tunnel: w436 -> [w446 w457]
                tunnel: w435 -> [w441 w452]
                frame True {
                  w449 = 0.0 ("element")
                  n132 = Build Array(w449, w450) -> (w444:dbl[])
                  n133 = Build Array(w448, w449) -> (w445:dbl[])
                  n134 = Add(x=w445, y=w446) -> (x+y=w442:dbl[])
                  n135 = Add(x=w442, y=w444) -> (x+y=w443:dbl[])
                  n136 = Insert Into Array(array=w451, new element #1=w441, new element #2=w442, new element #3=w443) -> (w447:dbl[][])  [unwired: 2 in]
                }
                frame False {
                  w460 = 0.0 ("element")
                  n137 = Build Array(w460, w461) -> (w456:dbl[])
                  n138 = Build Array(w459, w460) -> (w454:dbl[])
                  n139 = Add(x=w456, y=w457) -> (x+y=w455:dbl[])
                  n140 = Add(x=w455, y=w454) -> (x+y=w453:dbl[])
                  n141 = Insert Into Array(array=w462, new element #1=w452, new element #2=w455, new element #3=w453) -> (w458:dbl[][])  [unwired: 2 in]
                }
              }
            }
            frame True {
              w468 = 0.0 ("element")
              n142 = Subtract(x=w466, y=w463) -> (x-y=w467:dbl)
              n143 = Subtract(x=w465, y=w466) -> (x-y=w464:dbl)
              n144 = Build Array(w467, w468) -> (w479:dbl[])
              n145 = Build Array(w468, w469) -> (w477:dbl[])
              n146 = Build Array(w464, w468) -> (w471:dbl[])
              n147 = Add(x=w479, y=w473) -> (x+y=w478:dbl[])
              n148 = Add(x=w478, y=w477) -> (x+y=w472:dbl[])
              n149 = Add(x=w472, y=w471) -> (x+y=w470:dbl[])
              n150 = Insert Into Array(array=w475, new element #1=w474, new element #2=w478, new element #3=w472, new element #4=w470) -> (w476:dbl[][])  [unwired: 2 in]
            }
          }
          "Path out 2" <- w418
        }
      }
    }
  }
  n151 = Index Array(array=w97) -> (element=w88:T11)  [unwired: 1 in]
  n152 = call "SmoothPath.vi"("ignoreBall?"=w48, "AttackerAvoidArea"="AttackerAvoidArea", "ball"=w88, "defesa"=w85, "Initial State"="Initial Pos x,y", "Robot in"="Robot", "our_robots"=w90, "enemy_robots"=w89, "Path"=w25, "Goal"="Dest x,y") -> ("SmoothPath"=w87:dbl[][])  [unwired: 1 in]
  n153 = case shown="False" TRUE {
    tunnel: [w486 w487] -> w91
    tunnel: w90 -> [w485 _]
    tunnel: w89 -> [w484 _]
    tunnel: w88 -> [w483 _]
    tunnel: "Robot" -> [w482 _]
    tunnel: w87 -> [w481 w487]
    tunnel: w48 -> [w480 _]
    frame False {
      n154 = call "SmootherPath.vi"("ignoreBall?"=w480, "ball"=w483, "Robot in"=w482, "SmoothPath"=w481, "enemy_robots"=w484, "our_robots"=w485) -> ("SmootherPath"=w486:dbl[][])  [unwired: 5 in]
    }
    frame True {
    }
  }
  n155 = call "PrunePath.vi"("Robot in"="Robot", "Path in"=w91) -> ("Path out"=w28:dbl[][])  [unwired: 8 in, 1 out]
  n156 = feedback-in #1(w28) -> ()
  n157 = Select(t=w26, s=w1, f=w25) -> (s? t:f=→"Path":dbl[][])
  n158 = Select(t=w26, s=w1, f=w28) -> (s? t:f=→"Smooth Path":dbl[][])
